vi "Close.vi"(8 "error in (no error)":errorcluster, 11 "State in":T1={"State"=enum."Idle", "Start Time"=timestamp(0 s since 1904-01-01), "Configuration"={"DAQmx Task Name"="", "Output Channel"=0, "Time On (Sec)"=0.0, "Time Off (Sec)"=0.0, "Output Channel Names"=[], "Run?"=FALSE}, "Current Time"=timestamp(0 s since 1904-01-01), "First Iteration"=FALSE, "Data"={"D-O State"=enum."Off"}, "Process Name"="", "Output Error"=FALSE, "Log Started"=FALSE, "Cycle Period"=50.0} {"Configuration"."Output Channel" items=["Choose a Channel"]}) -> (0 "error out":errorcluster, 3 "State out":T1={"State"=enum."Idle", "Start Time"=timestamp(0 s since 1904-01-01), "Configuration"={"DAQmx Task Name"="", "Output Channel"=0, "Time On (Sec)"=0.0, "Time Off (Sec)"=0.0, "Output Channel Names"=[], "Run?"=FALSE}, "Current Time"=timestamp(0 s since 1904-01-01), "First Iteration"=FALSE, "Data"={"D-O State"=enum."Off"}, "Process Name"="", "Output Error"=FALSE, "Log Started"=FALSE, "Cycle Period"=50.0} {"Configuration"."Output Channel" items=["Choose a Channel"]})   [LabVIEW 2018, in "D-O Module.lvlib" / "D-O Module Engine.lvlib"]
uses:
  D-O Module Engine.lvlib
  Masterflex 7550-30/Masterflex 7550-30.lvlib
  Ismatec ISM 831C/Ismatec ISM 831C.lvlib
  Tacmina QI/Tacmina QI.lvlib
  VICI M50 Party Mode/VICI M6 M50 Party Mode.lvlib
  ASIA Pump.lvlib
  KNF Pump/KNF SIMDOS.lvlib
  State Enum.ctl
  D-O Module Settings Cluster.ctl
  D-O Module.lvlib
  State Cluster.ctl
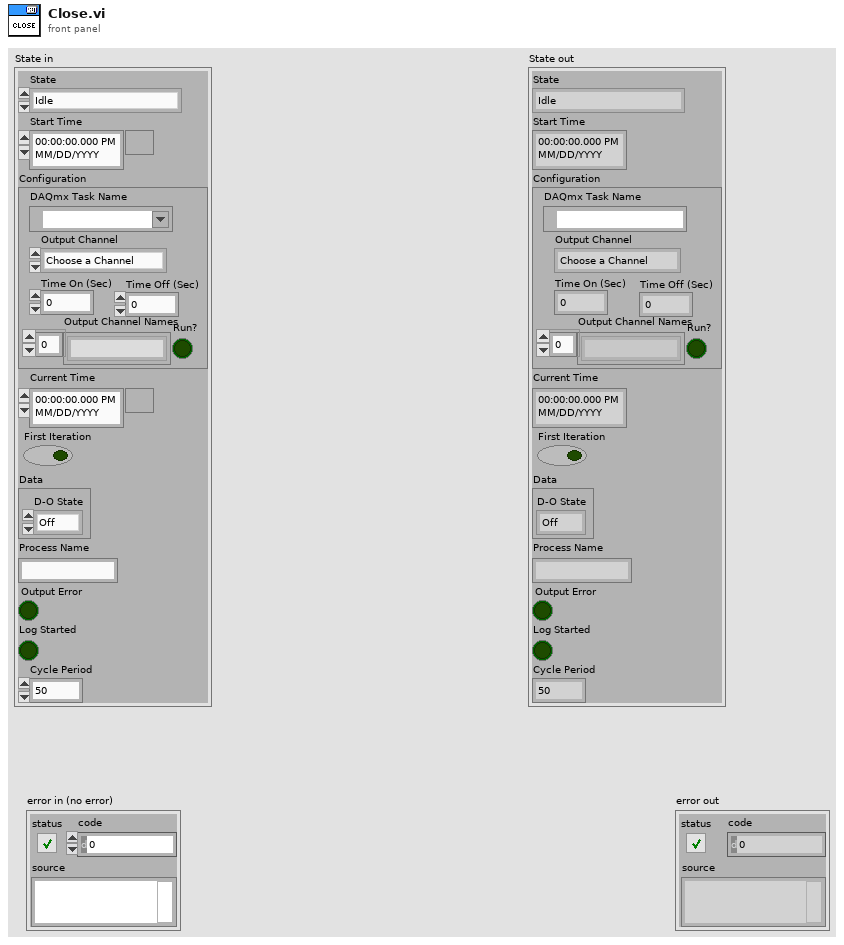
[diagram p1: front panel]
types:
  T1 = typedef "D-O Module.lvlib/D-O Module Engine.lvlib/State Cluster.ctl" = cluster{"State":T2, "Start Time":timestamp, "Configuration":T3, "Current Time":timestamp, "First Iteration":bool, "Data":cluster{"D-O State":enum16{"Off", "On", "Not Initialized"}}, "Process Name":string, "Output Error":bool, "Log Started":bool, "Cycle Period":dbl}
  T2 = typedef "D-O Module.lvlib/D-O Module Engine.lvlib/State Enum.ctl" = enum16{"Measuring", "Idle", "Paused"}
  T3 = typedef "D-O Module.lvlib/D-O Module Settings Cluster.ctl" = cluster{"DAQmx Task Name":refnum<k21>, "Output Channel":u16, "Time On (Sec)":dbl, "Time Off (Sec)":dbl, "Output Channel Names":string[], "Run?":bool}
  T4 = typedef "PID 2 Output Enum.ctl" = enum16{"Default", "Ismatec ISM 831C", "Masterflex 7550-30", "VICI M50", "Tacmina QI", "KNF SIMDOS", "ASIA Type C"}
  T5 = typedef "Masterflex 7550-30.lvlib/Settings Cluster.ctl" = cluster{"VISA resource name":refnum<visa-resource-name>, "Simulated?":bool, "Pump Number":dbl, "Reverse?":bool}
  T6 = typedef "Ismatec ISM 831C.lvlib/Ismatech Settings Cluster.ctl" = cluster{"VISA resource name":refnum<visa-resource-name>, "Simulated?":bool, "Pump Number":dbl, "Reverse?":bool}
  T7 = typedef "VICI M50 Party Mode.lvlib/Settings Cluster.ctl" = cluster{"VISA resource name":refnum<visa-resource-name>, "Simulated?":bool, "Pump Letter":string, "Reverse?":bool}
  T8 = typedef "Tacmina QI.lvlib/Tacmina QI DAQ Setting.ctl" = cluster{"Analog DAQ Task":refnum<k21>, "Digital DAQ Task":refnum<k21>}
  T9 = typedef "KNF SIMDOS.lvlib/Settings Cluster plus SIMDOS.ctl" = cluster{"VISA resource name":refnum<visa-resource-name>, "Simulated?":bool}
  T10 = typedef "ASIA Pump.lvlib/Pump Settings.ctl" = cluster{"ASIA Pump #":i32, "channel":i32, "Simulated":bool}
  T11 = typedef "VICI M6 M50 Party Mode.lvlib/Settings Cluster.ctl" = cluster{"VISA resource name":refnum<visa-resource-name>, "Simulated?":bool, "Pump Letter":string, "Reverse?":bool}
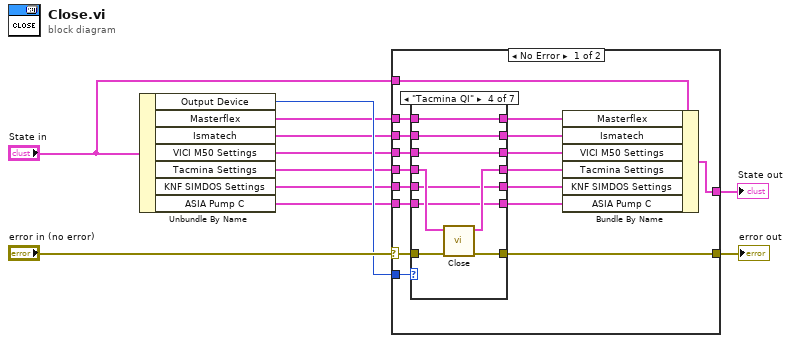
[diagram p0: block diagram]
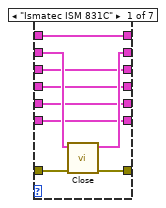
[diagram p2: hidden frame]
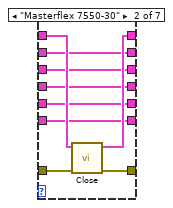
[diagram p3: hidden frame]
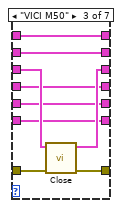
[diagram p4: hidden frame]
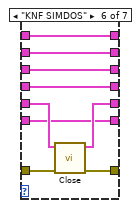
[diagram p6: hidden frame]
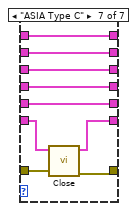
[diagram p7: hidden frame]
diagram:
  n1 = Unbundle By Name("State in") -> ("Output Device"=w7:T4, "Masterflex"=w6:T5, "Ismatech"=w5:T6, "VICI M50 Settings"=w4:T7, "Tacmina Settings"=w3:T8, "KNF SIMDOS Settings"=w2:T9, "ASIA Pump C"=w1:T10)
  n2 = case shown="No Error" "error in (no error)" {
    selector: "error in (no error)" -> [w22 w91]
    tunnel: [w25 w91] -> w10
    tunnel: "State in" -> [w28 w90]
    tunnel: [w27 w90] -> w8
    tunnel: w7 -> [w20 _]
    tunnel: w6 -> [w19 _]
    tunnel: w5 -> [w18 _]
    tunnel: w4 -> [w17 _]
    tunnel: w3 -> [w16 _]
    tunnel: w2 -> [w15 _]
    tunnel: w1 -> [w12 _]
    frame No Error {
      n3 = case shown="\"Tacmina QI\"" w20 {
        tunnel: w19 -> [w33 w46 w50 w61 w71 w76 w87]
        tunnel: [w33 w45 w50 w61 w71 w76 w87] -> w26
        tunnel: w18 -> [w35 w43 w51 w62 w67 w75 w86]
        tunnel: [w37 w44 w53 w63 w70 w79 w88] -> w25
        tunnel: w22 -> [w36 w42 w54 w64 w70 w80 w89]
        tunnel: [w34 w43 w51 w62 w67 w75 w86] -> w24
        tunnel: w17 -> [w32 w41 w55 w59 w69 w74 w85]
        tunnel: [w32 w41 w52 w59 w69 w74 w85] -> w23
        tunnel: w16 -> [w31 w40 w49 w58 w68 w73 w84]
        tunnel: [w31 w40 w49 w60 w68 w73 w84] -> w21
        tunnel: w15 -> [w30 w39 w47 w57 w65 w78 w83]
        tunnel: [w30 w39 w47 w57 w65 w77 w83] -> w14
        tunnel: [w29 w38 w48 w56 w66 w72 w81] -> w13
        tunnel: w12 -> [w29 w38 w48 w56 w66 w72 w82]
        frame "Ismatec ISM 831C" {
          n4 = call "Close.vi"("error in (no error)"=w36, "Ismatech Settings"=w35) -> ("error out"=w37:errorcluster, "Ismatech Settings"=w34:T6)  [unwired: 8 in]
        }
        frame "Masterflex 7550-30" {
          n5 = call "Close.vi"("error in (no error)"=w42, "Masterflex Settings in"=w46) -> ("error out"=w44:errorcluster, "Masterflex Settings out"=w45:T5)  [unwired: 8 in]
        }
        frame "VICI M50" {
          n6 = call "Close.vi"("error in (no error)"=w54, "VICI Settings"=w55) -> ("error out"=w53:errorcluster, "VICI Settings"=w52:T11)  [unwired: 8 in]
        }
        frame "Tacmina QI" {
          n7 = call "Close.vi"("error in"=w64, "Tacmina Settings in"=w58) -> ("error out"=w63:errorcluster, "Tacmina Settings out"=w60:T8)  [unwired: 8 in]
        }
        frame "Default", Default {
        }
        frame "KNF SIMDOS" {
          n8 = call "Close.vi"("error in (no error)"=w80, "KNF Settings"=w78) -> ("error out"=w79:errorcluster, "KNF Settings"=w77:T9)  [unwired: 8 in]
        }
        frame "ASIA Type C" {
          n9 = call "Close.vi"("error in (no error)"=w89, "ASIA Pump C"=w82) -> ("error out"=w88:errorcluster, "ASIA Pump C"=w81:T10)  [unwired: 7 in, 1 out]
        }
      }
      n10 = Bundle By Name(cluster=w28, "Masterflex"=w26, "Ismatech"=w24, "VICI M50 Settings"=w23, "Tacmina Settings"=w21, "KNF SIMDOS Settings"=w14, "ASIA Pump C"=w13) -> (w27:T1)
    }
    frame Error {
    }
  }
  "error out" <- w10
  "State out" <- w8
